vi "Display Biometry Average State Switch.vi"(11 "Switch":i32) -> (3 "State":T1)   [LabVIEW 2015, in "Utility VIs.lvlib"]
uses:
  Utility VIs.lvlib
  Browse/Support/Display Biometry Average State.ctl
  Browse/Browse.lvlib
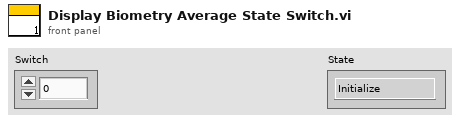
[diagram p1: front panel]
types:
  T1 = typedef "Browse.lvlib/Display Biometry Average State.ctl" = enum16{"Initialize", "Connect Database", "Display Biometry Ascan", "Display Biometry PD Image", "Display Biometry WTW Image", "Display Biometry Keratometric Image", "Update Biometry Average", "Wait For Event", "Exit"}
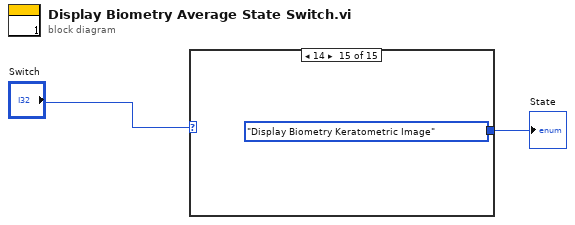
[diagram p0: block diagram]
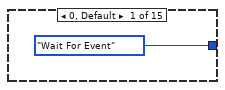
[diagram p2: hidden frame]
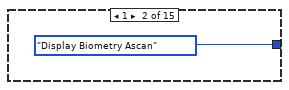
[diagram p3: hidden frame]
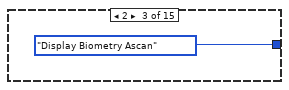
[diagram p4: hidden frame]
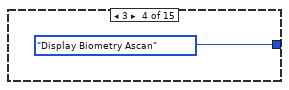
[diagram p5: hidden frame]
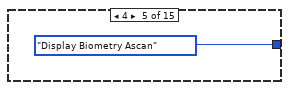
[diagram p6: hidden frame]
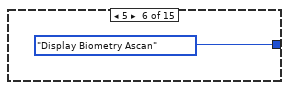
[diagram p7: hidden frame]
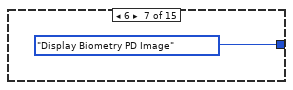
[diagram p8: hidden frame]
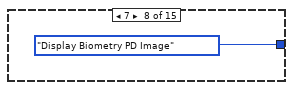
[diagram p9: hidden frame]
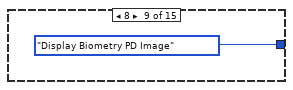
[diagram p10: hidden frame]
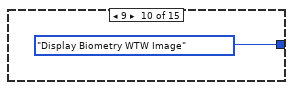
[diagram p11: hidden frame]
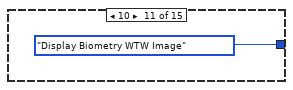
[diagram p12: hidden frame]
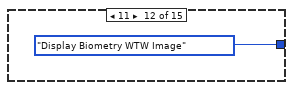
[diagram p13: hidden frame]
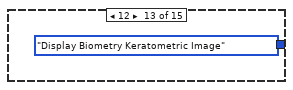
[diagram p14: hidden frame]
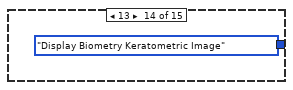
[diagram p15: hidden frame]
diagram:
  n1 = case shown="14" "Switch" {
    tunnel: [Display_Biometry_Average_State."Wait For Event" ("State") Display_Biometry_Average_State."Display Biometry Ascan" ("State") Display_Biometry_Average_State."Display Biometry Ascan" ("State") Display_Biometry_Average_State."Display Biometry Ascan" ("State") Display_Biometry_Average_State."Display Biometry Ascan" ("State") Display_Biometry_Average_State."Display Biometry Ascan" ("State") Display_Biometry_Average_State."Display Biometry PD Image" ("State") Display_Biometry_Average_State."Display Biometry PD Image" ("State") Display_Biometry_Average_State."Display Biometry PD Image" ("State") Display_Biometry_Average_State."Display Biometry WTW Image" ("State") Display_Biometry_Average_State."Display Biometry WTW Image" ("State") Display_Biometry_Average_State."Display Biometry WTW Image" ("State") Display_Biometry_Average_State."Display Biometry Keratometric Image" ("State") Display_Biometry_Average_State."Display Biometry Keratometric Image" ("State") Display_Biometry_Average_State."Display Biometry Keratometric Image" ("State")] -> w1
    frame 0, Default {
    }
    frame 1 {
    }
    frame 2 {
    }
    frame 3 {
    }
    frame 4 {
    }
    frame 5 {
    }
    frame 6 {
    }
    frame 7 {
    }
    frame 8 {
    }
    frame 9 {
    }
    frame 10 {
    }
    frame 11 {
    }
    frame 12 {
    }
    frame 13 {
    }
    frame 14 {
    }
  }
  "State" <- w1
